vi "ma_Convert Phase.vi"(9 "convert to degree (F)":bool, 10 "unwrap phase (F)":bool, 11 "phase (radian)":dbl[](array[numeric]) format="%0.2f") -> (3 "scaled phase":dbl[](array[numeric]) format="%0.2f")   [LabVIEW 2020, in "NI_MAPro.lvlib"]
uses:
  NI_MAPro.lvlib
  NI_AALPro.lvlib
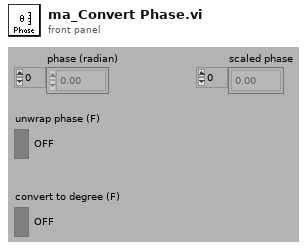
[diagram p1: front panel]
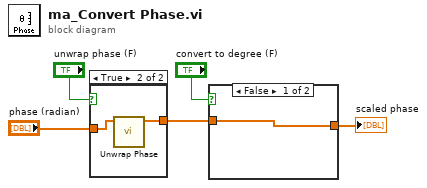
[diagram p0: block diagram]
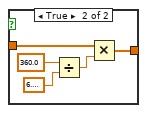
[diagram p3: hidden frame]
diagram:
  n1 = case shown="True" "unwrap phase (F)" {
    tunnel: "phase (radian)" -> [w6 w8]
    tunnel: [w6 w7] -> w2
    frame False {
    }
    frame True {
      n2 = call "Unwrap Phase.vi"("Phase"=w8) -> ("Unwrapped Phase"=w7:dbl[])  [unwired: 1 in, 9 out]
    }
  }
  n3 = case shown="False" "convert to degree (F)" {
    tunnel: [w9 w13] -> w5
    tunnel: w2 -> [w9 w14]
    frame False {
    }
    frame True {
      n4 = Divide(x=360.0, y=6.283185307179586) -> (x/y=w10:dbl)
      n5 = Multiply(x=w14, y=w10) -> (x*y=w13:dbl[])
    }
  }
  "scaled phase" <- w5
